vi "Boolean Case Structures.vi"() -> ()   [LabVIEW 2019]
panel:
  in  "Fahrenheit?":bool
  in  "stop":bool
  out "Temperature Output":dbl(slide) scale=0.0..212.0
  in  "Celsius Input":dbl(slide) scale=0.0..100.0
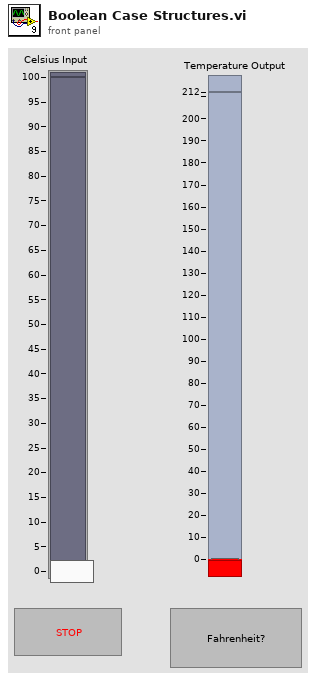
[diagram p1: front panel]
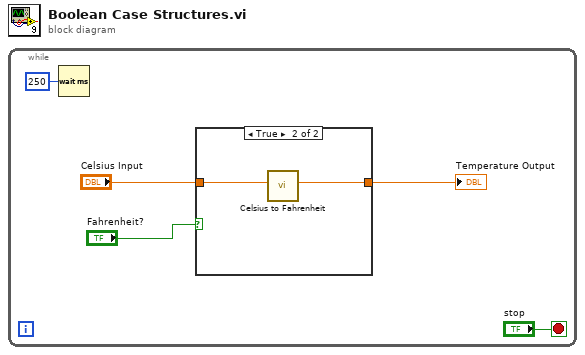
[diagram p0: block diagram]
diagram:
  n1 = while {
    stop <- "stop" stop-if-true
    n2 = Wait (ms)(milliseconds to wait=u32 250) -> ()  [unwired: 1 out]
    n3 = case shown="True" "Fahrenheit?" {
      tunnel: "Celsius Input" -> [w6 w8]
      tunnel: [w6 w7] -> w4
      frame False {
      }
      frame True {
        n4 = call "Celsius to Fahrenheit.vi"("Celsius"=w8) -> ("Fahrenheit"=w7:dbl)  [unwired: 10 in]
      }
    }
    "Temperature Output" <- w4
  }
